vi "Configurable Logging.vi"() -> ()   [LabVIEW 2018]
uses:
  src/api/logger_class/Log Levels.ctl
  src/api/logger_class/Logger.lvclass
  ff44e4a9-c346-414c-ae2a-efcf3ff82913.vi
  c9322c4e-9f12-43bd-adb9-b3674d2f7074.vi
  cbe71786-2e87-4bc7-85be-dae61289713f.vi
  593378fc-b3d1-4ba2-990a-aac09aa27d13.vi
  src/api/configuration/scopes/basic_scope/Basic.lvclass
  src/api/configuration/filters/regex_filter/Regex.lvclass
  src/api/configuration/handlers/file_handler/File Handler.lvclass
  src/api/configuration/formatters/format_string_formatter/Format String.lvclass
  src/api/configuration/filters/regex_filter/New (Element).vi
  src/api/configuration/scopes/basic_scope/New (Element).vi
panel:
  out "ms timer":u32[](array[numeric])
  out "elapsed time":u32[](array[numeric])
  out "iterations":i32[](array[numeric])
  in  "error in (no error)":errorcluster
  out "error out":errorcluster
  in  "total iterations":i32=30
  # "Locals"
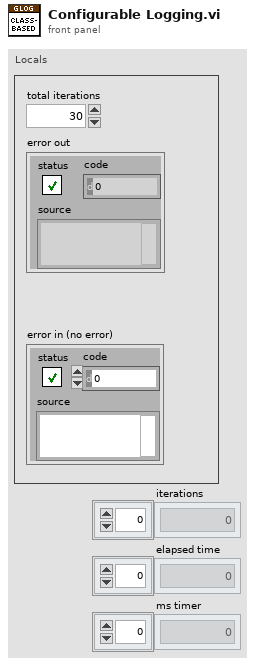
[diagram p1: front panel]
types:
  T1 = typedef "GLog.lvlib/Logger.lvclass/Log Levels.ctl" = enum16{"Trace", "Debug", "Info", "Warning", "Error", "Critical"}
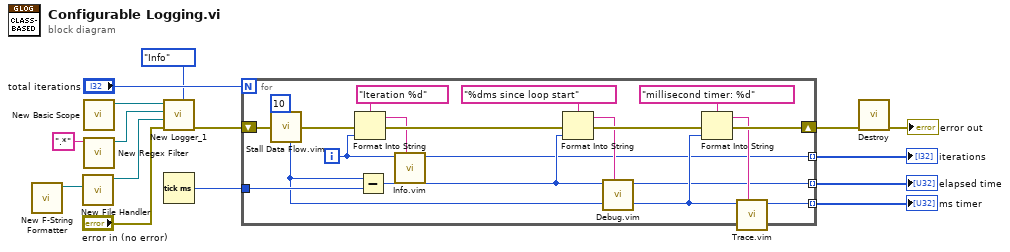
[diagram p0: block diagram]
diagram:
  n1 = call "New F-String Formatter.vi"() -> ("new f-string formatter"=w2:refnum<class "Format String.lvclass">)  [unwired: 11 in]
  n2 = call "New File Handler.vi"("formatter (JSON)"=w2) -> ("file handler"=w3:refnum<class "File Handler.lvclass">)  [unwired: 10 in]
  n3 = call-poly "New Basic Scope.vi"() -> ("basic scope"=w5:refnum<class "Basic.lvclass">)  [unwired: 11 in]
  n4 = call-poly "New Regex Filter.vi"("regex string"=".*") -> ("regex out"=w4:refnum<class "Regex.lvclass">)  [unwired: 9 in, 1 out]
  n5 = call "New Logger_1.vi"("minimum log level (Info)"=Log_Levels."Info" ("minimum log level"), "error in (no error)"="error in (no error)", "log handler (file handler)"=w3, "log filter (none)"=w4, "logger scope (all)"=w5) -> ("error out"=w6:errorcluster)  [unwired: 5 in, 1 out]
  n6 = Tick Count (ms)() -> (millisecond timer value=w15:u32)
  n7 = for {
    N: "total iterations" -> [_]
    tunnel: w15 -> [w34]
    shift-right: [w27] -> w13
    shift-left: w6 -> [w20]
    tunnel: [w18] -> w11 mode=indexing
    tunnel: [w17] -> w10 mode=indexing
    tunnel: [w16] -> w9 mode=indexing
    i -> [w26]
    n8 = call "Stall Data Flow.vim"("value in"=w20, "milliseconds to wait"=u32 10 ("loop iteration delay [ms]")) -> ("millisecond timer value"=w22:u32, "value out"=w19:errorcluster)
    n9 = Format Into String(format string="Iteration %d" ("message"), error in=w19, w26) -> (resulting string=w25:string, error out=w29:errorcluster)  [unwired: 1 in]
    n10 = Subtract(x=w22, y=w34) -> (x-y=w23:u32)
    n11 = call "Info.vim"("data in (null)"=w26, "message"=w25) -> ("data out"=w18:i32)  [unwired: 9 in]
    n12 = Format Into String(format string="%dms since loop start" ("message"), error in=w29, w23) -> (resulting string=w24:string, error out=w28:errorcluster)  [unwired: 1 in]
    n13 = call "Debug.vim"("data in (null)"=w23, "message"=w24) -> ("data out"=w17:u32)  [unwired: 9 in]
    n14 = Format Into String(format string="millisecond timer: %d" ("message"), error in=w28, w22) -> (resulting string=w21:string, error out=w27:errorcluster)  [unwired: 1 in]
    n15 = call "Trace.vim"("data in (null)"=w22, "message"=w21) -> ("data out"=w16:u32)  [unwired: 9 in]
  }
  "iterations" <- w11
  "elapsed time" <- w10
  "ms timer" <- w9
  n16 = call "Destroy.vi"("error in (no error)"=w13) -> ("error out"=→"error out":errorcluster)  [unwired: 9 in, 1 out]
